vi "TurnLeftRight.vi"(6 "Timeout (ms)":u32=2000, 7 "Start time":u32, 10 "Degrees":dbl=10.0 format="%#_13g", 11 "Left/Right":enum16{"Left", "Right", ""}(ring)) -> (3 "Done":bool)   [LabVIEW 2013]
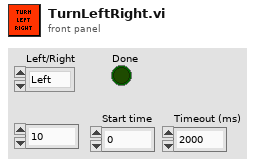
[diagram p1: front panel]
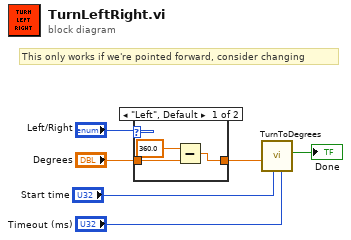
[diagram p0: block diagram]
diagram:
  # "This only works if we're pointed forward, consider changing"
  n1 = case shown="\"Left\", Default" "Left/Right" {
    tunnel: [w9 w10] -> w4
    tunnel: "Degrees" -> [w8 w10]
    frame "Left", Default {
      n2 = Subtract(x=360.0, y=w8) -> (x-y=w9:dbl)
    }
    frame "Right" {
    }
  }
  n3 = call "TurnToDegrees.vi"("Timeout (ms)"="Timeout (ms)", "Start time"="Start time", "Degrees"=w4) -> ("Done"=→"Done":bool)  [unwired: 6 in, 2 out]
